vi "generator1 (SubVI).vi"(6 "Amp":dbl, 7 "Numeric":dbl, 9 "phase":dbl, 10 "freq":dbl, 11 "Sygnal":T1(ring)) -> (3 "Gaussian white noise":dbl)   [LabVIEW 2025]
uses:
  <vilib>/ptbypt/NI_PtbyPt.lvlib
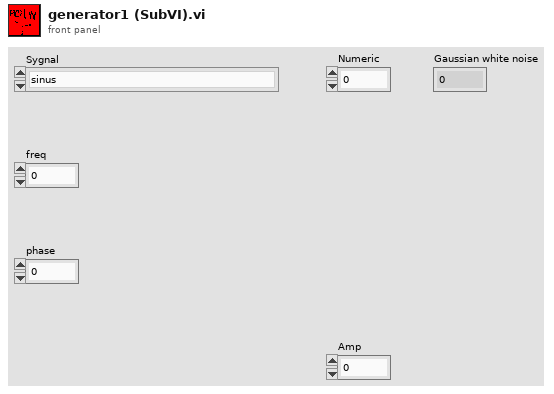
[diagram p1: front panel]
types:
  T1 = enum16{"sinus", "prostokat", "pila", "trojkat", "rozklad losowy", "rozklad normalny"}
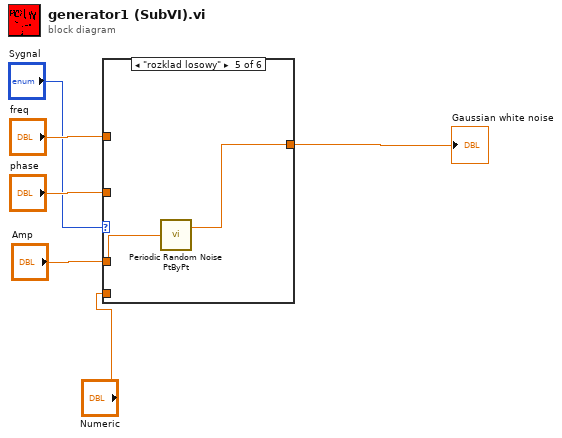
[diagram p0: block diagram]
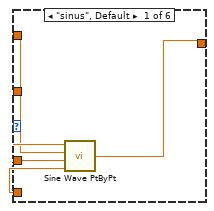
[diagram p2: hidden frame]
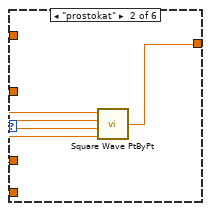
[diagram p3: hidden frame]
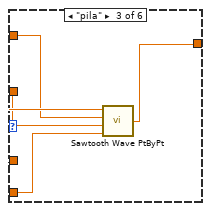
[diagram p4: hidden frame]
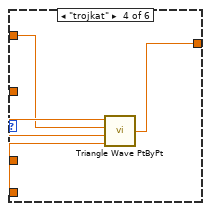
[diagram p5: hidden frame]
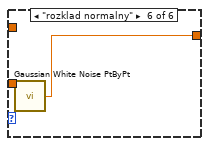
[diagram p6: hidden frame]
diagram:
  n1 = case shown="\"rozklad losowy\"" "Sygnal" {
    tunnel: [w11 w16 w21 w26 w28 w29] -> w2
    tunnel: "Amp" -> [w10 w12 w20 w25 w27 _]
    tunnel: "freq" -> [w9 w15 w19 w24 _ _]
    tunnel: "phase" -> [w8 w14 w18 w22 _ _]
    tunnel: "Numeric" -> [w7 w13 w17 w23 _ _]
    frame "sinus", Default {
      n2 = call <vilib>:"Sine Wave PtByPt.vi"("time"=w7, "phase"=w8, "frequency"=w9, "amplitude"=w10) -> ("sine wave"=w11:dbl)
    }
    frame "prostokat" {
      n3 = call <vilib>:"Square Wave PtByPt.vi"("amplitude"=w12, "frequency"=w15, "phase"=w14, "time"=w13) -> ("square wave"=w16:dbl)  [unwired: 1 in]
    }
    frame "pila" {
      n4 = call <vilib>:"Sawtooth Wave PtByPt.vi"("time"=w17, "phase"=w18, "frequency"=w19, "amplitude"=w20) -> ("sawtooth wave"=w21:dbl)
    }
    frame "trojkat" {
      n5 = call <vilib>:"Triangle Wave PtByPt.vi"("time"=w23, "phase"=w22, "frequency"=w24, "amplitude"=w25) -> ("triangle wave"=w26:dbl)
    }
    frame "rozklad losowy" {
      n6 = call <vilib>:"Periodic Random Noise PtByPt.vi"("spectral amplitude"=w27) -> ("periodic random noise"=w28:dbl)  [unwired: 3 in, 1 out]
    }
    frame "rozklad normalny" {
      n7 = call <vilib>:"Gaussian White Noise PtByPt.vi"() -> ("Gaussian white noise"=w29:dbl)  [unwired: 3 in]
    }
  }
  "Gaussian white noise" <- w2
